vi "Set Class Instance.vi"(11 "OsciloscopeType":string) -> (3 "specific class reference":refnum<class "Generador.lvclass">)   [LabVIEW 2020, in "FGen.lvlib"]
uses:
  FGen.lvlib
  Generador/Generador.lvclass
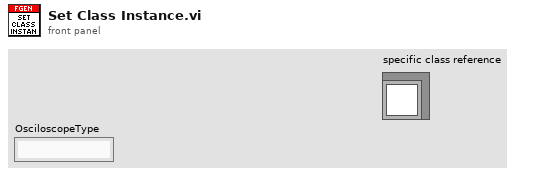
[diagram p1: front panel]
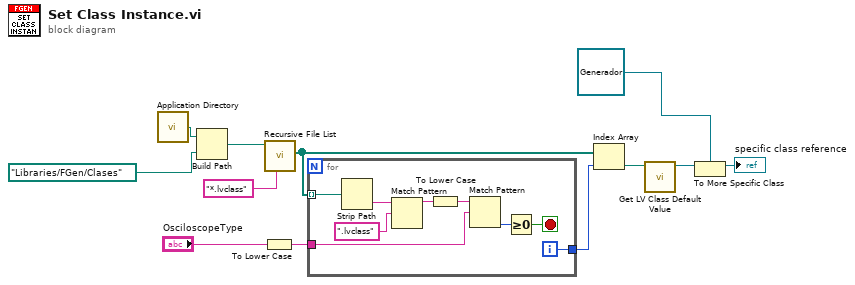
[diagram p0: block diagram]
diagram:
  n1 = call <vilib>:"Application Directory.vi"() -> ("Application Directory"=w12:path)
  n2 = Build Path(base path=w12, name or relative path=path "Libraries/FGen/Clases") -> (appended path=w11:path)
  n3 = To Lower Case(string="OsciloscopeType") -> (all lower case string=w7:string)
  n4 = call <vilib>:"Recursive File List.vi"("pattern"="*.lvclass", "Folder Path"=w11) -> ("All Files in Dir"=w6:path[])  [unwired: 5 in, 4 out]
  n5 = for {
    tunnel: w6 -> [w16] mode=indexing
    tunnel: w7 -> [w21]
    tunnel: [w17] -> w5
    i -> [w17]
    stop <- w18 stop-if-true
    n6 = Strip Path(path=w16) -> (name=w15:string)  [unwired: 1 out]
    n7 = Match Pattern(string=w15, regular expression=".lvclass") -> (before substring=w13:string)  [unwired: 1 in, 3 out]
    n8 = To Lower Case(string=w13) -> (all lower case string=w20:string)
    n9 = Match Pattern(string=w20, regular expression=w21) -> (offset past match=w19:i32)  [unwired: 1 in, 3 out]
    n10 = Greater Or Equal To 0?(x=w19) -> (x >= 0?=w18:bool)
  }
  n11 = Index Array(array=w6, index=w5) -> (element=w4:path)
  n12 = call <vilib>:"Get LV Class Default Value.vi"("class path"=w4) -> ("object"=w9:refnum<class>)  [unwired: 9 in, 1 out]
  n13 = To More Specific Class(target class=refnum<class "Generador.lvclass"> refnum ("FGen.lvlib:Generator"), reference=w9) -> (specific class reference=→"specific class reference":refnum<class "Generador.lvclass">)  [unwired: 1 in, 1 out]
